vi "Update FF_I.vi"(0 "source adress PID out":u32, 1 "source adress e(n)":u32, 2 "destination adress":u32, 3 "Buffer size":u32, 5 "input valid":bool=TRUE, 7 "a0":fxp<+/-,32,2>, 8 "Disable e(n)":bool, 9 "b0":fxp<+/-,32,2>, 10 "Reset":bool=TRUE, 11 "cavity filter - a":fxp<+/-,32,4>, 13 "cavity filter - b":fxp<+/-,32,17>) -> (19 "output valid":bool)   [LabVIEW 2018]
uses:
  <vilib>/rvi/Emulation/niFpgaSctlEmulationGetInTimedLoop.vi
  <vilib>/rvi/Memory/Memory_Emulation/nirvimemoryFastEmulation.vi
  <vilib>/rvi/Memory/Memory_Emulation/nirvimemoryEmulation.vi
  <vilib>/rvi/Emulation/niFpgaEmulationIsFPGAContextNoSignature.vi
  <vilib>/rvi/DataTransferAndStorage/Container/Common/niFpgaContainerGetUniqueNameForEmu.vi
  <vilib>/rvi/Emulation/niFpgaProcessEmulError.vi
  <vilib>/rvi/errors/nirviReportUnexpectedCaseInternalError (U32).vi
  <vilib>/rvi/DataTransferAndStorage/Container/XNode/niFpgaContainer.xnode
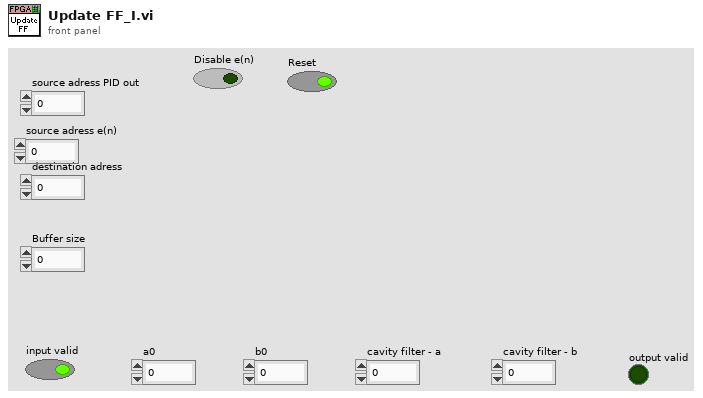
[diagram p1: front panel]
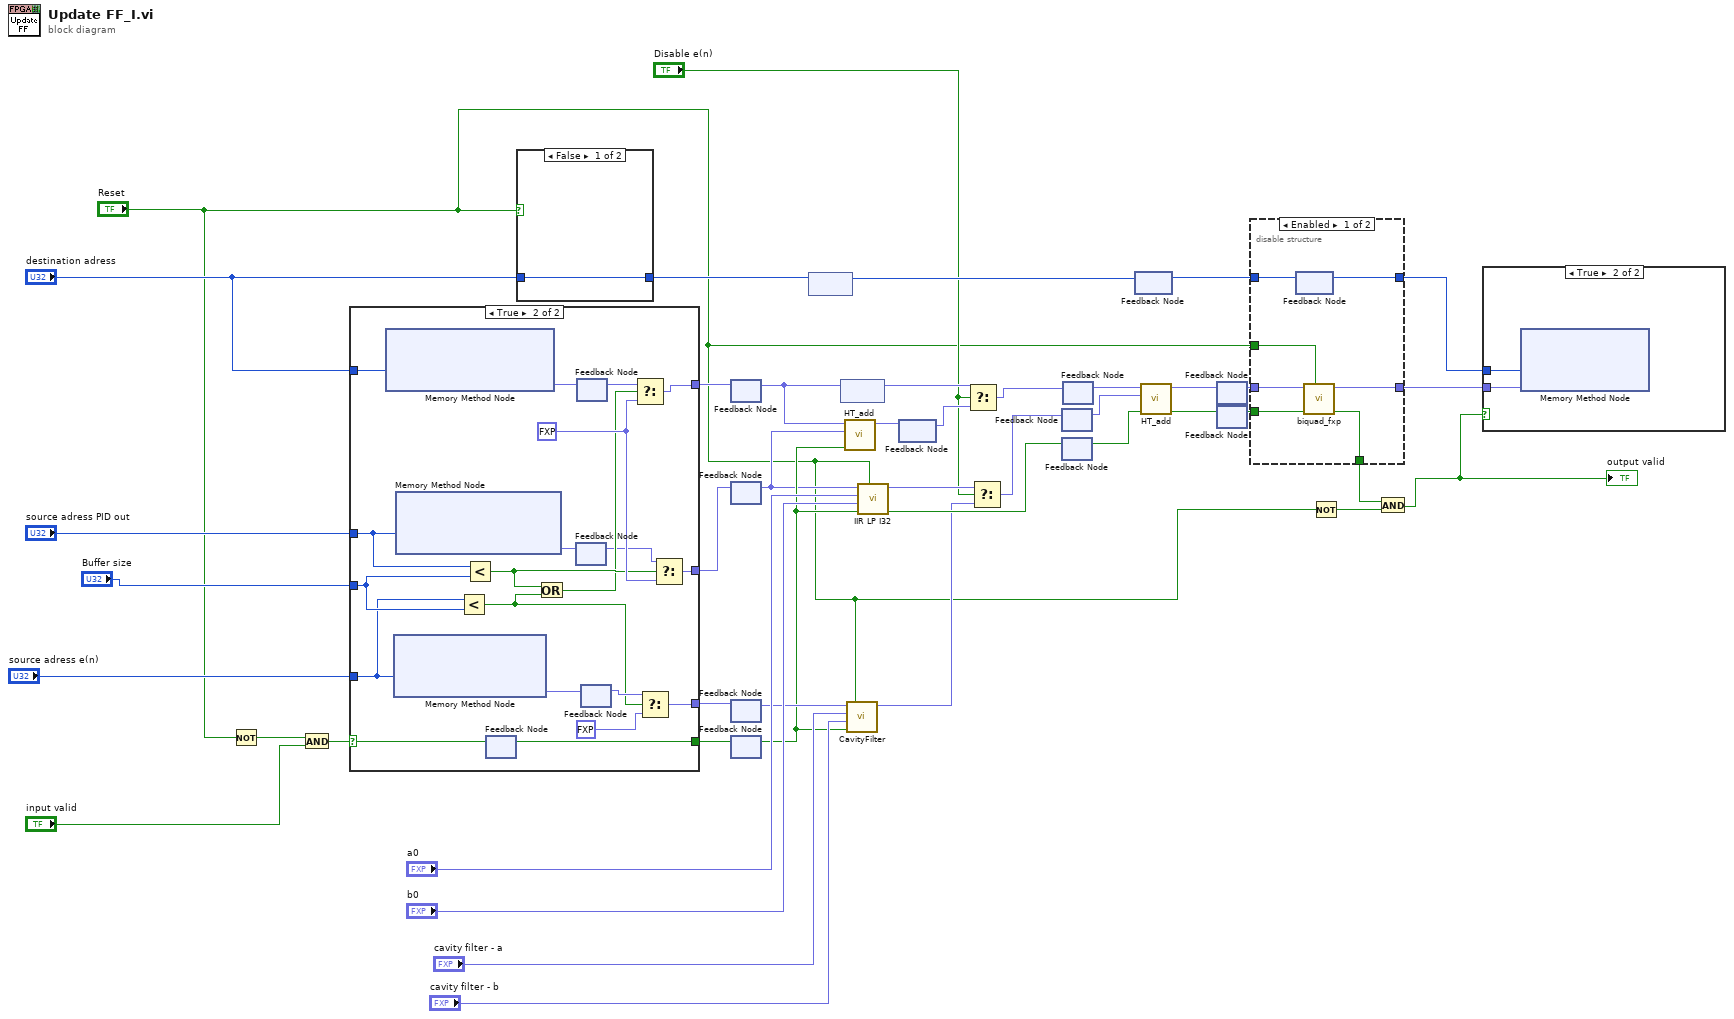
[diagram p0: block diagram]
diagram:
  n1 = Not(x="Reset") -> (.not. x?=w32:bool)
  n2 = And(x=w32, y="input valid") -> (x .and. y?=w33:bool)
  n3 = case shown="True" w33 {
    selector: w33 -> [_ w62]
    tunnel: [_ w58] -> w42
    tunnel: "source adress PID out" -> [_ w60]
    tunnel: [_ w56] -> w41
    tunnel: "destination adress" -> [_ w64]
    tunnel: [_ w61] -> w38
    tunnel: "Buffer size" -> [_ w54]
    tunnel: "source adress e(n)" -> [_ w53]
    tunnel: [_ w49] -> w16
    frame False {
    }
    frame True {
      w55 = fxp<+/-,32,14> 0.0 ("f")
      n4 = xnode ("Memory Method Node")("Address"=w64) -> ("Data"=w63:fxp<+/-,32,14>)  [unwired: 1 in, 1 out]
      n5 = xnode ("Memory Method Node")("Address"=w53) -> ("Data"=w52:fxp<+/-,32,14>)  [unwired: 1 in, 1 out]
      n6 = xnode ("Memory Method Node")("Address"=w60) -> ("Data"=w59:fxp<+/-,32,14>)  [unwired: 1 in, 1 out]
      n7 = Less?(x=w53, y=w54) -> (x < y?=w47:bool)
      n8 = Less?(x=w60, y=w54) -> (x < y?=w48:bool)
      n9 = feedback #1() -> (w61:bool)  [unwired: 1 in]
      n10 = feedback-in #1(w62) -> ()
      n11 = Or(x=w48, y=w47) -> (x .or. y?=w46:bool)
      n12 = feedback #2() -> (w45:fxp<+/-,32,14>)  [unwired: 1 in]
      n13 = feedback-in #2(w59) -> ()
      n14 = feedback #3() -> (w57:fxp<+/-,32,14>)  [unwired: 1 in]
      n15 = feedback-in #3(w63) -> ()
      n16 = feedback #4() -> (w51:fxp<+/-,32,14>)  [unwired: 1 in]
      n17 = feedback-in #4(w52) -> ()
      n18 = Select(t=w57, s=w46, f=w55) -> (s? t:f=w56:fxp<+/-,32,14>)
      n19 = Select(t=w51, s=w47, f=fxp<+/-,32,14> 0.0) -> (s? t:f=w49:fxp<+/-,32,14>)
      n20 = Select(t=w45, s=w48, f=w55) -> (s? t:f=w58:fxp<+/-,32,14>)
    }
  }
  n21 = case shown="False" "Reset" {
    tunnel: "destination adress" -> [w65 _]
    tunnel: [w65 _] -> w39
    frame False {
    }
    frame True {
    }
  }
  n22 = feedback #5() -> (w12:fxp<+/-,32,14>)  [unwired: 1 in]
  n23 = feedback-in #5(w41) -> ()
  n24 = feedback-in #6(w42) -> ()
  n25 = feedback #6() -> (w10:fxp<+/-,32,14>)  [unwired: 1 in]
  n26 = feedback #7() -> (w15:fxp<+/-,32,14>)  [unwired: 1 in]
  n27 = feedback-in #7(w16) -> ()
  n28 = feedback #8() -> (w11:bool)  [unwired: 1 in]
  n29 = feedback-in #8(w38) -> ()
  n30 = feedback #9() -> (w22:u32)  [unwired: 1 in]
  n31 = feedback-in #9(w39) -> ()
  n32 = feedback #10() -> (w8:fxp<+/-,32,14>)  [unwired: 1 in]
  n33 = feedback-in #10(w12) -> ()
  n34 = call "HT_add.vi"("input valid"=w11, "y"=w10, "x"=w12) -> ("x+y"=w9:fxp<+/-,32,14>)  [unwired: 7 in, 1 out]
  n35 = call "CavityFilter.vi"("Reset"="Reset", "input valid"=w11, "b"="cavity filter - b", "a"="cavity filter - a", "Value in"=w15) -> ("Value out"=w4:fxp<+/-,32,14>)  [unwired: 5 in, 1 out]
  n36 = call "IIR LP I32.vi"("Reset"="Reset", "input valid"=w11, "b0"="b0", "a0"="a0", "Value in"=w10) -> ("output valid"=w24:bool, "Value out"=w5:fxp<+/-,32,14>)  [unwired: 5 in]
  n37 = feedback #11() -> (w6:fxp<+/-,32,14>)  [unwired: 1 in]
  n38 = feedback-in #11(w9) -> ()
  n39 = Select(t=w8, s="Disable e(n)", f=w6) -> (s? t:f=w7:fxp<+/-,32,14>)
  n40 = Select(t=w5, s="Disable e(n)", f=w4) -> (s? t:f=w3:fxp<+/-,32,14>)
  n41 = feedback #12() -> (w26:fxp<+/-,32,14>)  [unwired: 1 in]
  n42 = feedback-in #12(w3) -> ()
  n43 = feedback #13() -> (w29:bool)  [unwired: 1 in]
  n44 = feedback-in #13(w24) -> ()
  n45 = feedback #14() -> (w23:fxp<+/-,32,14>)  [unwired: 1 in]
  n46 = feedback-in #14(w7) -> ()
  n47 = feedback #15() -> (w18:u32)  [unwired: 1 in]
  n48 = feedback-in #15(w22) -> ()
  n49 = call "HT_add.vi"("input valid"=w29, "y"=w26, "x"=w23) -> ("output valid"=w27:bool, "x+y"=w28:fxp<+/-,32,14>)  [unwired: 7 in]
  n50 = feedback #16() -> (w21:fxp<+/-,32,14>)  [unwired: 1 in]
  n51 = feedback-in #16(w28) -> ()
  n52 = feedback #17() -> (w20:bool)  [unwired: 1 in]
  n53 = feedback-in #17(w27) -> ()
  n54 = disable-structure shown="Enabled" {
    disable-tunnel: [w72 w74] -> w31
    disable-tunnel: [w71 w75] -> w30
    disable-tunnel: "Reset" -> [w70 _]
    disable-tunnel: w21 -> [w69 w74]
    disable-tunnel: w20 -> [w68 w73]
    disable-tunnel: [w67 w73] -> w19
    disable-tunnel: w18 -> [w66 w75]
    frame Enabled {
      n55 = feedback #18() -> (w71:u32)  [unwired: 1 in]
      n56 = feedback-in #18(w66) -> ()
      n57 = call "biquad_fxp.vi"("reset"=w70, "input valid"=w68, "x"=w69) -> ("output valid"=w67:bool, "y"=w72:fxp<+/-,32,14>)  [unwired: 7 in]
    }
    frame Disabled {
    }
  }
  n58 = Not(x="Reset") -> (.not. x?=w25:bool)
  n59 = And(x=w19, y=w25) -> (x .and. y?=w37:bool)
  "output valid" <- w37
  n60 = case shown="True" w37 {
    tunnel: w31 -> [_ w77]
    tunnel: w30 -> [_ w76]
    frame False {
    }
    frame True {
      n61 = xnode ("Memory Method Node")("Address"=w76, "Data"=w77) -> ()  [unwired: 1 in, 1 out]
    }
  }
